vi "PID Gain Schedule (DBL Array).vi"(4 "PID gain schedule":T2(array[cluster])=[{"PID gains"={"proportional gain (Kc)"=1.0, "integral time (Ti, min)"=0.01, "derivative time (Td, min)"=0.0}, "max value"=100.0}] {"max value" format="%.2f"; "PID gains"."derivative time (Td, min)" format="%.3f"; "PID gains"."integral time (Ti, min)" format="%.3f"; "PID gains"."proportional gain (Kc)" format="%.3f"}, 5 "gain scheduling value":dbl[](array[numeric])=[0.0] format="%.2f") -> (1 "PID gains out":T1(array[cluster]) {"derivative time (Td, min)" format="%.3f"; "integral time (Ti, min)" format="%.3f"; "proportional gain (Kc)" format="%.3f"}, 2 "index out":i32[](array[numeric]))   [LabVIEW 2020, in "NI_PID_pid.lvlib"]
doc: "Selects a set of PID gains from a gain schedule for the control of processes that require different sets of gains for different regions of operation, such as highly nonlinear processes. Use the DBL instance of this VI to implement a single control loop. Use the DBL Array instance to implement parallel multi-loop control."
uses:
  NI_PID_pid.lvlib
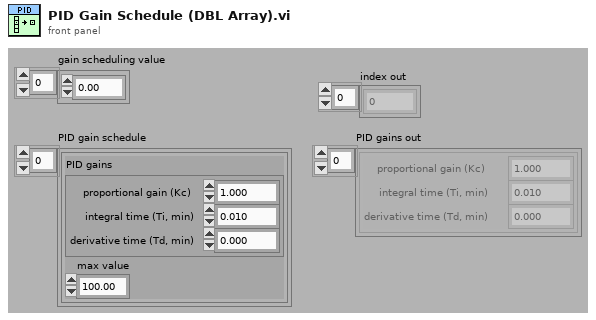
[diagram p1: front panel]
types:
  T1 = cluster{"proportional gain (Kc)":dbl, "integral time (Ti, min)":dbl, "derivative time (Td, min)":dbl}[]
  T2 = cluster{"PID gains":cluster{"proportional gain (Kc)":dbl, "integral time (Ti, min)":dbl, "derivative time (Td, min)":dbl}, "max value":dbl}[]
  T3 = cluster{"proportional gain (Kc)":dbl, "integral time (Ti, min)":dbl, "derivative time (Td, min)":dbl}
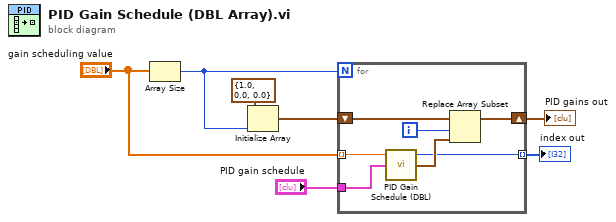
[diagram p0: block diagram]
diagram:
  n1 = Array Size(array="gain scheduling value") -> (size(s)=w2:i32)
  n2 = Initialize Array(T3 {"proportional gain (Kc)"=1.0, "integral time (Ti, min)"=0.0, "derivative time (Td, min)"=0.0} ("PID gains out"), w2) -> (w4:T1)
  n3 = for {
    N: w2 -> [_]
    shift-right: [w14] -> w5
    shift-left: w4 -> [w9]
    tunnel: "gain scheduling value" -> [w12] mode=indexing
    tunnel: "PID gain schedule" -> [w11]
    tunnel: [w8] -> w1 mode=indexing
    i -> [w10]
    n4 = call "PID Gain Schedule (DBL).vi"("PID gain schedule"=w11, "gain scheduling value"=w12) -> ("PID gains out"=w13:T3, "index out"=w8:i32)  [unwired: 2 out]
    n5 = Replace Array Subset(array=w9, new element=w13, index=w10) -> (w14:T1)
  }
  "PID gains out" <- w5
  "index out" <- w1
